vi "GenStepProf.vi"() -> ()   [LabVIEW 2016]
panel:
  out "size(s)":i32
  out "Z":dbl[](graph)
  out "Y":dbl[](graph)
  out "X":dbl[](graph)
  out "Input RUY":T1
  in  "No Cycles":i32=3
  in  "Dwell Time [s]":dbl=2.0
  in  "Step Size [deg or mm]":dbl=0.5
  in  "Select Joint No.":T2(ring)=enum."Joint 3"
  out "Joint 4 Graph":dbl[](graph)
  out "Joint 3 Graph":dbl[](graph)
  out "Joint 2 Graph":dbl[](graph)
  out "Joint 1 Graph":dbl[](graph)
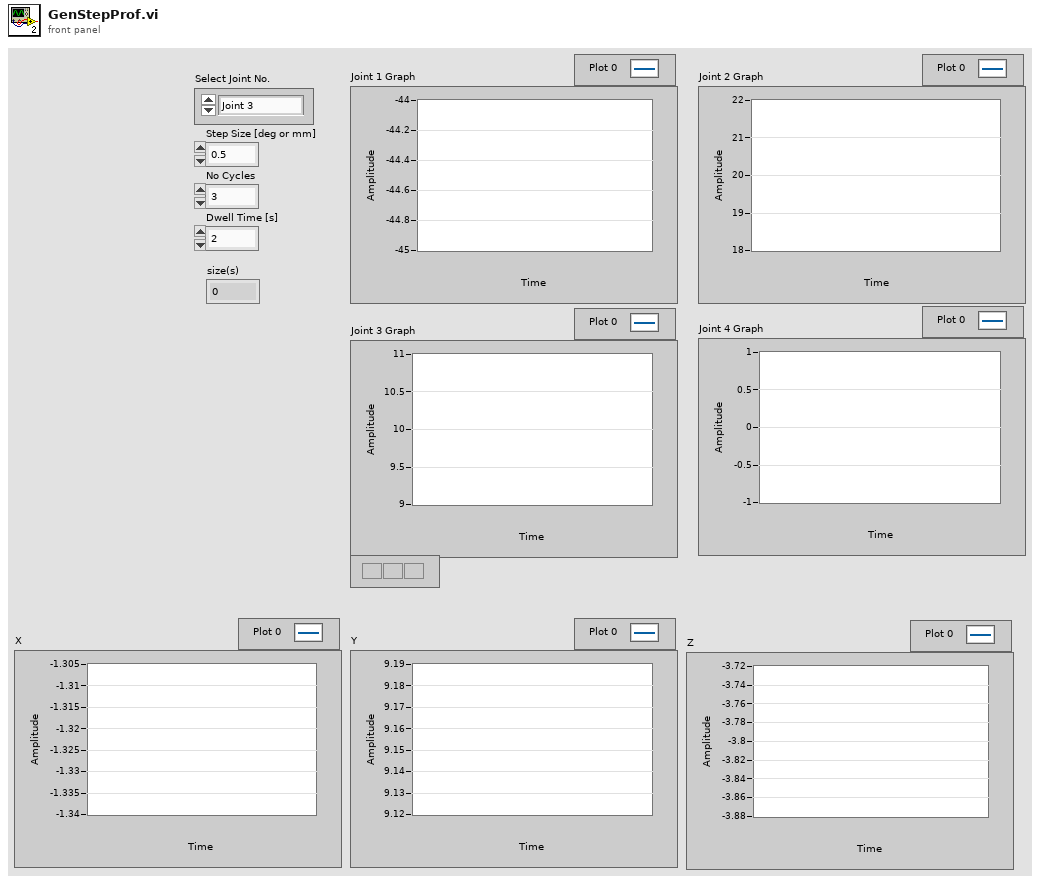
[diagram p1: front panel]
types:
  T1 = cluster{"Ref":cluster{"theta 1 Array":dbl[], "theta 2 Array":dbl[], "d3 Array":dbl[], "theta 4 Array":dbl[]}, "uFF":cluster{"theta 1 Array":dbl[], "theta 2 Array":dbl[], "d3 Array":dbl[], "theta 4 Array":dbl[]}, "yOut":cluster{"theta 1 Array":dbl[], "theta 2 Array":dbl[], "d3 Array":dbl[], "theta 4 Array":dbl[]}}
  T2 = enum16{"Joint 1", "Joint 2", "Joint 3", "Joint 4"}
  T3 = cluster{"theta 1 Array":dbl[], "theta 2 Array":dbl[], "d3 Array":dbl[], "theta 4 Array":dbl[]}
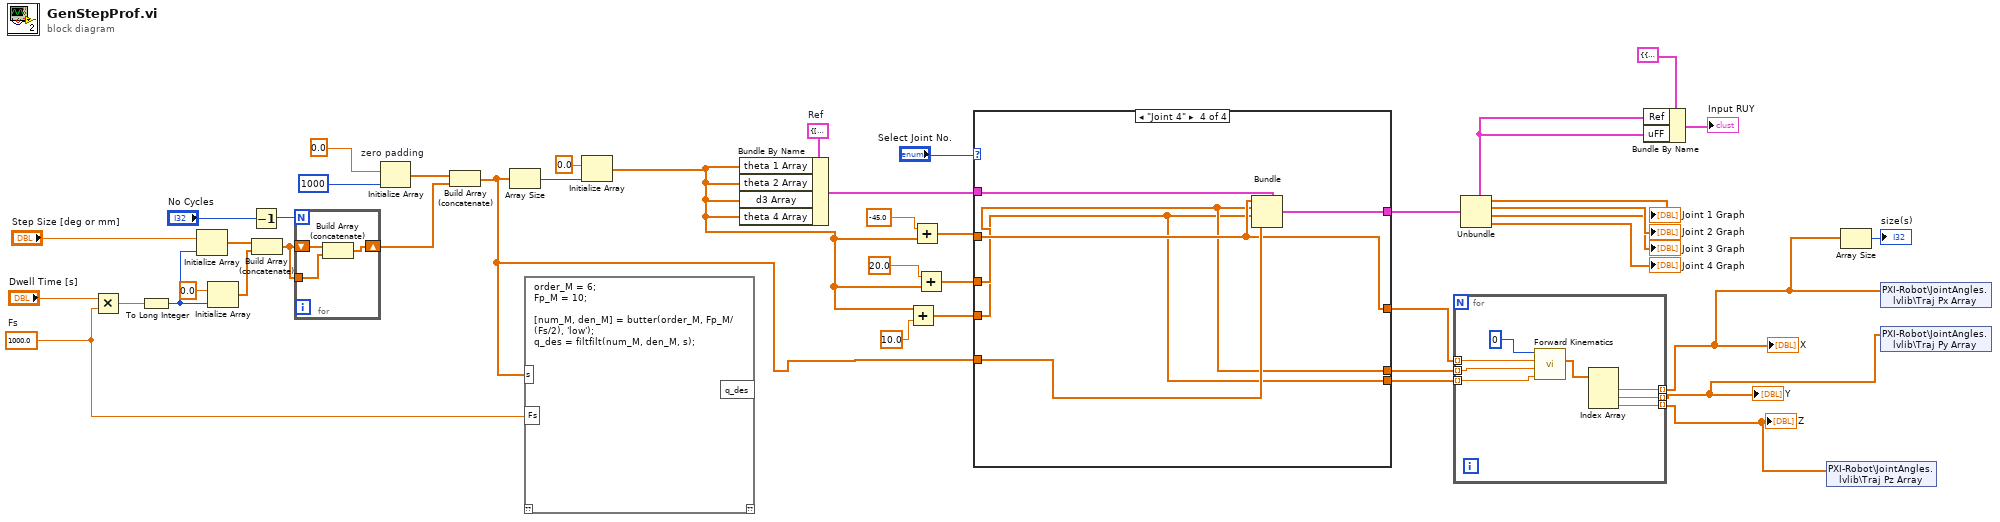
[diagram p0: block diagram]
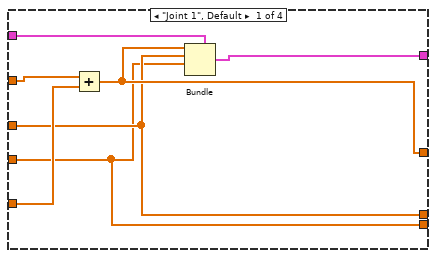
[diagram p2: hidden frame]
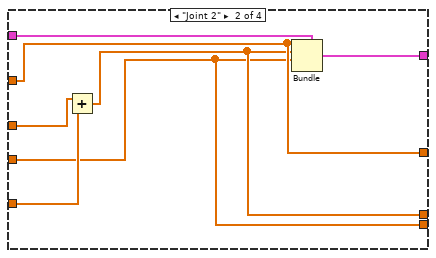
[diagram p3: hidden frame]
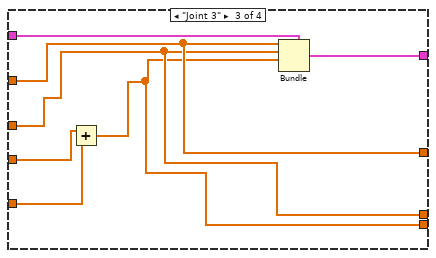
[diagram p4: hidden frame]
diagram:
  w29 = T3 {"theta 1 Array"=[], "theta 2 Array"=[], "d3 Array"=[], "theta 4 Array"=[]}  # Ref
  w18 = 1000.0  # Fs
  n1 = Multiply(x="Dwell Time [s]", y=w18) -> (x*y=w40:dbl)
  n2 = To Long Integer(number=w40) -> (32bit integer=w39:i32)
  n3 = Initialize Array("Step Size [deg or mm]", w39) -> (w36:dbl[])
  n4 = Initialize Array(0.0 ("element"), w39) -> (w37:dbl[])
  n5 = Decrement(x="No Cycles") -> (x-1=w33:i32)
  n6 = Build Array (concatenate)(w36, w37) -> (w35:dbl[])
  n7 = for {
    N: w33 -> [_]
    shift-right: [w44] -> w22
    shift-left: w35 -> [w45]
    tunnel: w35 -> [w43]
    n8 = Build Array (concatenate)(w45, w43) -> (w44:dbl[])
  }
  n9 = Initialize Array "zero padding"(0.0 ("element"), 1000 ("dimension size")) -> (w23:dbl[])
  n10 = Build Array (concatenate)(w23, w22) -> (w11:dbl[])
  n11 = Array Size(array=w11) -> (size(s)=w32:i32)
  n12 = script code="order_M = 6;\nFp_M = 10;\n\n[num_M, den_M] = butter(order_M, Fp_M/(Fs/2), 'low');\nq_des = filtfilt(num_M, den_M, s);"("s"=w11, "Fs"=w18) -> ()  [unwired: 1 in, 2 out]
  n13 = Initialize Array(0.0 ("element"), w32) -> (w12:dbl[])
  n14 = Bundle By Name(cluster=w29, "theta 1 Array"=w12, "theta 2 Array"=w12, "d3 Array"=w12, "theta 4 Array"=w12) -> (w20:T3)
  n15 = Add(x=w12, y=10.0) -> (x+y=w10:dbl[])
  n16 = Add(x=-45.0, y=w12) -> (x+y=w16:dbl[])
  n17 = Add(x=20.0, y=w12) -> (x+y=w9:dbl[])
  n18 = case shown="\"Joint 4\"" "Select Joint No." {
    tunnel: w20 -> [w52 w59 w66 w72]
    tunnel: w11 -> [w49 w56 w63 w71]
    tunnel: [w51 w58 w65 w70] -> w15
    tunnel: w16 -> [w50 w55 w62 w69]
    tunnel: w10 -> [w46 w53 w64 w67]
    tunnel: w9 -> [w47 w57 w61 w68]
    tunnel: [w48 w55 w62 w69] -> w7
    tunnel: [w47 w54 w61 w68] -> w6
    tunnel: [w46 w53 w60 w67] -> w5
    frame "Joint 1", Default {
      n19 = Add(x=w50, y=w49) -> (x+y=w48:dbl[])
      n20 = Bundle(cluster=w52, "theta 1 Array"=w48, "theta 2 Array"=w47, "d3 Array"=w46) -> (w51:T3)  [unwired: 1 in]
    }
    frame "Joint 2" {
      n21 = Add(x=w57, y=w56) -> (x+y=w54:dbl[])
      n22 = Bundle(cluster=w59, "theta 1 Array"=w55, "theta 2 Array"=w54, "d3 Array"=w53) -> (w58:T3)  [unwired: 1 in]
    }
    frame "Joint 3" {
      n23 = Add(x=w64, y=w63) -> (x+y=w60:dbl[])
      n24 = Bundle(cluster=w66, "theta 1 Array"=w62, "theta 2 Array"=w61, "d3 Array"=w60) -> (w65:T3)  [unwired: 1 in]
    }
    frame "Joint 4" {
      n25 = Bundle(cluster=w72, "theta 1 Array"=w69, "theta 2 Array"=w68, "d3 Array"=w67, "theta 4 Array"=w71) -> (w70:T3)
    }
  }
  n26 = for {
    tunnel: w7 -> [w79] mode=indexing
    tunnel: w6 -> [w78] mode=indexing
    tunnel: w5 -> [w77] mode=indexing
    tunnel: [w75] -> w2 mode=indexing
    tunnel: [w74] -> w4 mode=indexing
    tunnel: [w73] -> w3 mode=indexing
    n27 = call "Forward Kinematics.vi"("j3"=w77, "j2"=w78, "j1"=w79, "armID"=0) -> ("XYZ Out Array"=w76:dbl[])  [unwired: 7 in]
    n28 = Index Array(array=w76) -> (element #1=w75:dbl, element #2=w74:dbl, element #3=w73:dbl)  [unwired: 3 in]
  }
  "X" <- w2
  "Y" <- w4
  "Z" <- w3
  n29 = Unbundle(w15) -> ("theta 1 Array"=→"Joint 1 Graph":dbl[], "theta 2 Array"=→"Joint 2 Graph":dbl[], "d3 Array"=→"Joint 3 Graph":dbl[], "theta 4 Array"=→"Joint 4 Graph":dbl[])
  n30 = Bundle By Name(cluster=T1 {"Ref"={"theta 1 Array"=[], "theta 2 Array"=[], "d3 Array"=[], "theta 4 Array"=[]}, "uFF"={"theta 1 Array"=[], "theta 2 Array"=[], "d3 Array"=[], "theta 4 Array"=[]}, "yOut"={"theta 1 Array"=[], "theta 2 Array"=[], "d3 Array"=[], "theta 4 Array"=[]}} ("Input RUY"), "Ref"=w15, "uFF"=w15) -> (→"Input RUY":T1)
  n31 = shared-variable "PXI-Robot\\JointAngles.lvlib\\Traj Pz Array"(w3) -> ()  [unwired: 1 in, 1 out]
  n32 = Array Size(array=w2) -> (size(s)=→"size(s)":i32)
  n33 = shared-variable "PXI-Robot\\JointAngles.lvlib\\Traj Px Array"(w2) -> ()  [unwired: 1 in, 1 out]
  n34 = shared-variable "PXI-Robot\\JointAngles.lvlib\\Traj Py Array"(w4) -> ()  [unwired: 1 in, 1 out]
